vi "BRig_Host__Loop_Consumer_RunState__closedLoop_parseOutput2_thres.vi"(11 "String":string) -> (1 "output_thres2":u16, 2 "output_thres1":u16, 3 "output_thres":bool)   [LabVIEW 2014]
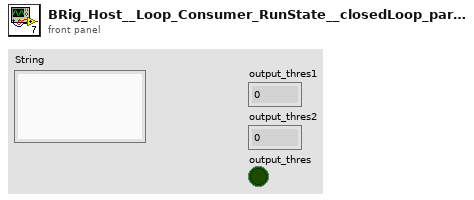
[diagram p1: front panel]
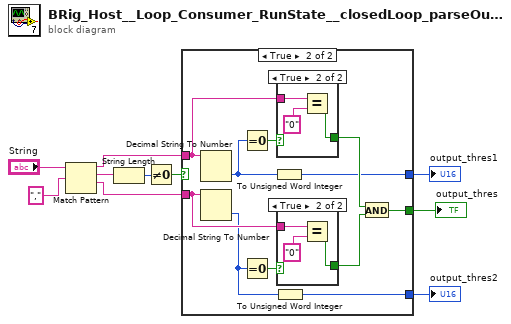
[diagram p0: block diagram]
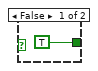
[diagram p3: hidden frame]
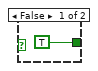
[diagram p4: hidden frame]
diagram:
  n1 = Match Pattern(string="String", regular expression=",") -> (before substring=w5:string, match substring=w7:string, after substring=w4:string)  [unwired: 1 in, 1 out]
  n2 = String Length(string=w7) -> (length=w8:i32)
  n3 = Not Equal To 0?(x=w8) -> (x != 0?=w6:bool)
  n4 = case shown="True" w6 {
    tunnel: w5 -> [_ w20]
    tunnel: w4 -> [_ w18]
    tunnel: [_ w13] -> w3
    tunnel: [_ w11] -> w2
    tunnel: [_ w15] -> w1
    frame False {
    }
    frame True {
      n5 = Decimal String To Number(string=w20) -> (number=w14:i32)  [unwired: 2 in, 1 out]
      n6 = Decimal String To Number(string=w18) -> (number=w12:i32)  [unwired: 2 in, 1 out]
      n7 = Equal To 0?(x=w14) -> (x = 0?=w21:bool)
      n8 = Equal To 0?(x=w12) -> (x = 0?=w19:bool)
      n9 = To Unsigned Word Integer(number=w14) -> (unsigned 16bit integer=w13:u16)
      n10 = To Unsigned Word Integer(number=w12) -> (unsigned 16bit integer=w11:u16)
      n11 = case shown="True" w21 {
        tunnel: w20 -> [_ w27]
        tunnel: [TRUE w29] -> w17
        frame False {
        }
        frame True {
          n12 = Equal?(x=w27, y="0" ("x")) -> (x = y?=w29:bool)
        }
      }
      n13 = case shown="True" w19 {
        tunnel: w18 -> [_ w23]
        tunnel: [TRUE w25] -> w16
        frame False {
        }
        frame True {
          n14 = Equal?(x=w23, y="0" ("x")) -> (x = y?=w25:bool)
        }
      }
      n15 = And(x=w17, y=w16) -> (x .and. y?=w15:bool)
    }
  }
  "output_thres1" <- w3
  "output_thres2" <- w2
  "output_thres" <- w1
